vi "Get Sciscan FOV.vi"(8 "error in":errorcluster, 11 "GFG Refnum":refnum<vi>) -> (0 "error out":errorcluster, 2 "FOV":cluster{"Width [um]":dbl, "Height [um]":dbl}={"Width [um]"=400.0, "Height [um]"=400.0}, 3 "GFG Refnum Out":refnum<vi>)   [LabVIEW 2012, in "Sciscan Scope Daemon.lvlib"]
uses:
  Sciscan Scope Daemon.lvlib
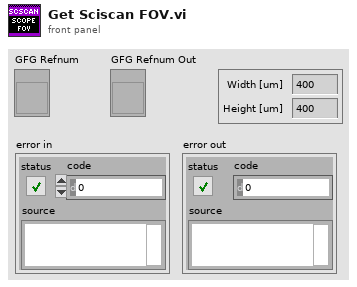
[diagram p1: front panel]
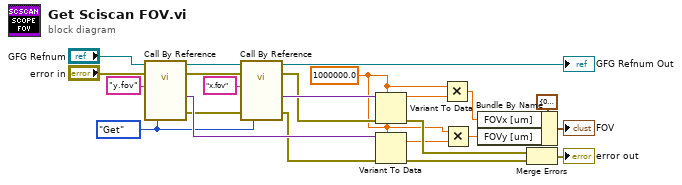
[diagram p0: block diagram]
diagram:
  w1 = 1000000.0
  w19 = enum16{"Init", "Set", "Get"}."Get" ("Action")
  n1 = call-by-ref "?"(reference="GFG Refnum", error in="error in", "Variable Name in"="y.fov", "Action"=w19) -> (reference out=w23:refnum<vi>, error out=w22:errorcluster, "Variant Out"=w21:variant, 19:"error out"=w16:errorcluster)  [unwired: 11 in, 5 out]
  n2 = call-by-ref "?"(reference=w23, error in=w22, "Variable Name in"="x.fov", 5:"error in (no error)"=w16, "Action"=w19) -> (reference out=→"GFG Refnum Out":refnum<vi>, error out=w13:errorcluster, "Variant Out"=w20:variant, 19:"error out"=w12:errorcluster)  [unwired: 10 in, 5 out]
  n3 = Variant To Data(error in=w13, type=w1, Variant=w20) -> (data=w5:dbl, error out=w10:errorcluster)
  n4 = Variant To Data(error in=w12, type=w1, Variant=w21) -> (data=w2:dbl, error out=w11:errorcluster)
  n5 = Multiply(x=w1, y=w5) -> (x*y=w4:dbl)
  n6 = Multiply(x=w1, y=w2) -> (x*y=w3:dbl)
  n7 = Bundle By Name(cluster=cluster{"FOVx [um]":dbl, "FOVy [um]":dbl} {"FOVx [um]"=0.0, "FOVy [um]"=0.0} ("FOV"), "FOVx [um]"=w4, "FOVy [um]"=w3) -> (→"FOV":cluster{"FOVx [um]":dbl, "FOVy [um]":dbl})
  n8 = Merge Errors(w10, w11) -> (→"error out":errorcluster)
